vi "ConvertDataDoubleToFloat.vi"(8 "error in (no error)":errorcluster, 10 "Double In":dbl[](array[numeric]), 11 "controller in":refnum<k24>) -> (0 "error out":errorcluster, 2 "Float Out":sgl[](array[numeric]), 3 "controller out":refnum<k24>)   [LabVIEW 2010]
uses:
  c:/aerotech/controller/stable/a3200/pc/labview/2010/bin/Aerotech.A3200.dll
  bin/Aerotech.A3200.dll
  c:/aerotech/controller/stable/a3200/pc/labview/2010/bin/Aerotech.A3200.LabVIEW.dll
  bin/Aerotech.A3200.LabVIEW.dll
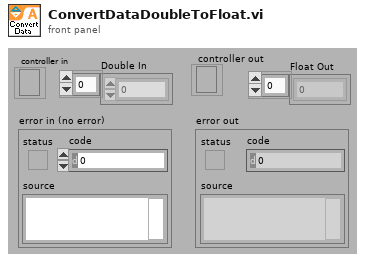
[diagram p1: front panel]
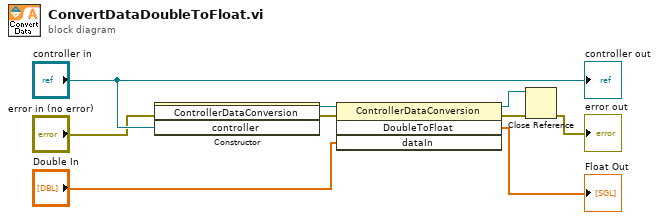
[diagram p0: block diagram]
diagram:
  n1 = constructor class="ControllerDataConversion"(error in="error in (no error)", "controller"="controller in") -> (reference out=w9:refnum<k24>, error out=w6:errorcluster)  [unwired: 2 in, 2 out]
  n2 = invoke class="ControllerDataConversion" method="DoubleToFloat"(reference=w9, error in=w6, "dataIn"="Double In") -> (reference out=w4:refnum<k24>, error out=w3:errorcluster, "DoubleToFloat"=→"Float Out":sgl[])  [unwired: 1 in, 1 out]
  n3 = Close Reference(reference=w4, error in (no error)=w3) -> (error out=→"error out":errorcluster)
  "controller out" <- "controller in"
